vi "Field_Sweep_AMI.vi"   [LabVIEW 2016]
uses:
  Global/Global Variables/global.vi
  Global/Global Variables/Data_Display_global.vi
types:
  T1 = enum16{"", "RAMPING", "HOLDING", "PAUSED", "MANUAL UP", "MANUAL DOWN", "ZEROING CURRENT", "QUENCH DETECTED", "HEATING SWITCH", "AT ZER0", "COOLING SWITCH"}
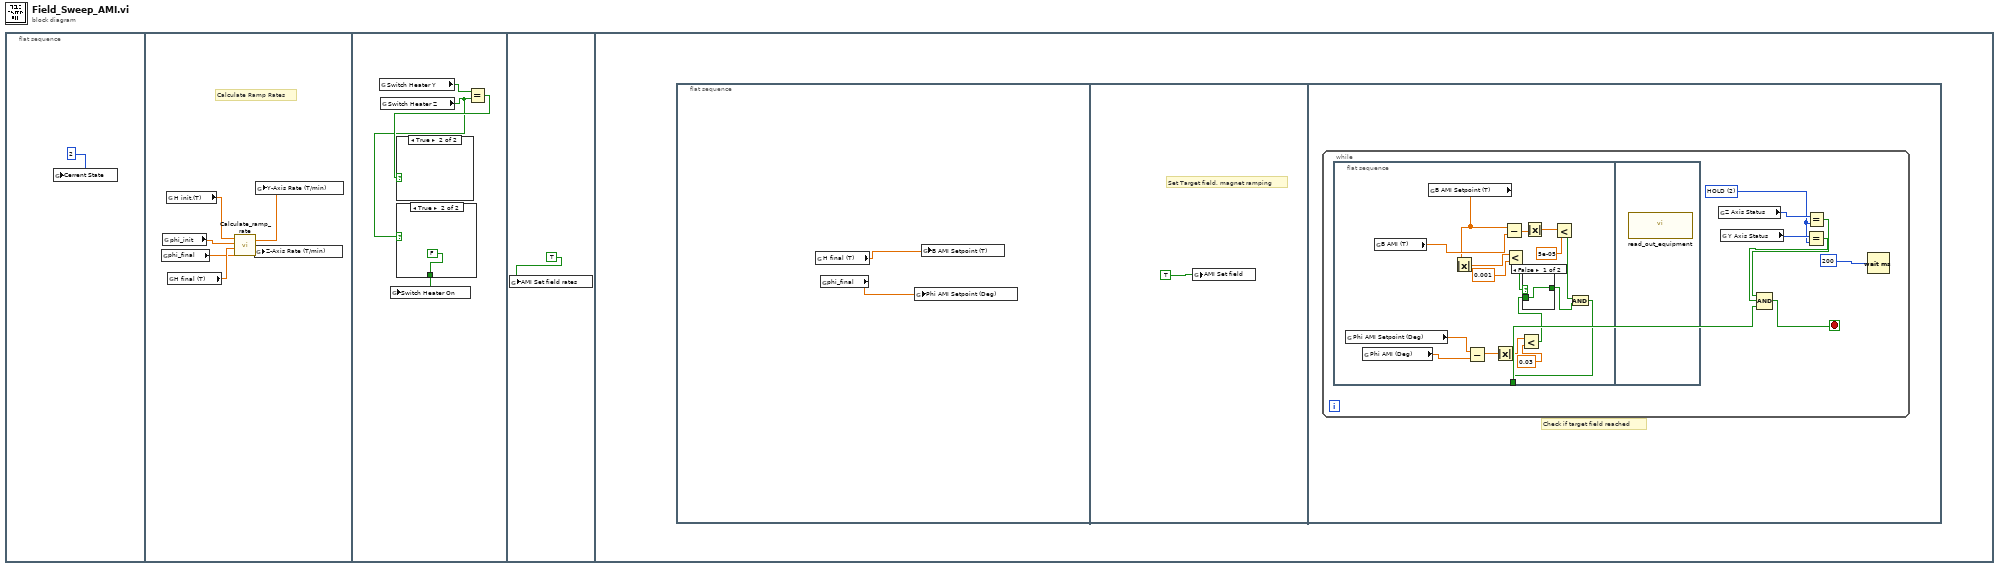
[diagram p0: block diagram]
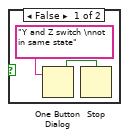
[diagram p2: hidden frame]
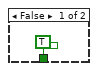
[diagram p3: hidden frame]
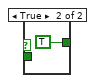
[diagram p4: hidden frame]
diagram:
  n1 = flat-sequence {
    frame #0 {
      n2 = global write "global.vi" "Cerrent State"(2) -> ()
    }
    frame #1 {
      # "Calculate Ramp Rates"
      n3 = global read "global.vi" "phi_final"() -> (w2:dbl)
      n4 = global read "global.vi" "phi_init"() -> (w3:dbl)
      n5 = global read "global.vi" "H init.(T)"() -> (w4:dbl)
      n6 = global read "global.vi" "H final (T)"() -> (w5:dbl)
      n7 = call "Calculate_ramp_rate.vi"("Phi (Deg)"=w2, "H_final (T)"=w5, "Phi_init (Deg)"=w3, "H_init (T)"=w4) -> ("Z-Ramp"=w6:dbl, "Y-Ramp"=w7:dbl)  [unwired: 2 in]
      n8 = global write "Data_Display_global.vi" "Z-Axis Rate (T/min)"(w6) -> ()
      n9 = global write "Data_Display_global.vi" "Y-Axis Rate (T/min)"(w7) -> ()
    }
    frame #2 {
      n10 = global read "Data_Display_global.vi" "Switch Heater Y"() -> (w10:bool)
      n11 = global read "Data_Display_global.vi" "Switch Heater Z"() -> (w8:bool)
      n12 = case shown="True" w8 {
        tunnel: [TRUE FALSE] -> w11
        frame False {
        }
        frame True {
        }
      }
      n13 = global write "Data_Display_global.vi" "Switch Heater On"(w11) -> ()
      n14 = Equal?(x=w10, y=w8) -> (x = y?=w9:bool)
      n15 = case shown="True" w9 {
        frame False {
          n16 = One Button Dialog(message="Y and Z switch \nnot in same state") -> (true=w12:bool)  [unwired: 1 in]
          n17 = Stop(stop? (T)=w12) -> ()
        }
        frame True {
        }
      }
    }
    frame #3 {
      n18 = global write "Data_Display_global.vi" "AMI Set field rates"(TRUE) -> ()
    }
    frame #4 {
      n19 = flat-sequence {
        frame #0 {
          n20 = global read "global.vi" "H final (T)"() -> (w18:dbl)
          n21 = global read "global.vi" "phi_final"() -> (w17:dbl)
          n22 = global write "Data_Display_global.vi" "Phi AMI Setpoint (Deg)"(w17) -> ()
          n23 = global write "Data_Display_global.vi" "B AMI Setpoint (T)"(w18) -> ()
        }
        frame #1 {
          # "Set Target field, magnet ramping"
          n24 = global write "Data_Display_global.vi" "AMI Set field"(TRUE) -> ()
        }
        frame #2 {
          # "Check if target field reached"
          n25 = while {
            stop <- w21 stop-if-true
            w20 = u16 2 items=["RAMP"=1, "HOLD"=2, "Paused"=3, "Manual Up"=4, "Manual Down"=5, "Zeroing Current"=6, "Quench Detected"=7, "At Zero"=8, "Heating Switch"=9, "Cooling Switch "=10] ("Ramping Mode")
            n26 = flat-sequence {
              tunnel: [w34] -> w22
              frame #0 {
                n27 = global read "Data_Display_global.vi" "Phi AMI Setpoint (Deg)"() -> (w37:dbl)
                n28 = global read "Data_Display_global.vi" "Phi AMI (Deg)"() -> (w36:dbl)
                n29 = global read "Data_Display_global.vi" "B AMI (T)"() -> (w41:dbl)
                n30 = global read "Data_Display_global.vi" "B AMI Setpoint (T)"() -> (w30:dbl)
                n31 = Absolute Value(x=w30) -> (abs(x)=w33:dbl)
                n32 = Subtract(x=w37, y=w36) -> (x-y=w38:dbl)
                n33 = Absolute Value(x=w38) -> (abs(x)=w39:dbl)
                n34 = Subtract(x=w30, y=w41) -> (x-y=w43:dbl)
                n35 = Less?(x=w33, y=0.001) -> (x < y?=w31:bool)
                n36 = Less?(x=w39, y=0.03) -> (x < y?=w29:bool)
                n37 = case shown="False" w31 {
                  tunnel: [w45 TRUE] -> w28
                  tunnel: w29 -> [w45 _]
                  frame False {
                  }
                  frame True {
                  }
                }
                n38 = Absolute Value(x=w43) -> (abs(x)=w42:dbl)
                n39 = Less?(x=w42, y=5e-05) -> (x < y?=w35:bool)
                n40 = And(x=w35, y=w28) -> (x .and. y?=w34:bool)
              }
              frame #1 {
                n41 = call "read_out_equipment.vi"() -> ()  [unwired: 1 in]
              }
            }
            n42 = global read "Data_Display_global.vi" "Z Axis Status"() -> (w26:T1)
            n43 = global read "Data_Display_global.vi" "Y Axis Status"() -> (w25:T1)
            n44 = Equal?(x=w25, y=w20) -> (x = y?=w23:bool)
            n45 = Equal?(x=w26, y=w20) -> (x = y?=w24:bool)
            n46 = Compound Arithmetic op=AND(w24, w23, w22) -> (w21:bool)
            n47 = Wait (ms)(milliseconds to wait=200) -> ()  [unwired: 1 out]
          }
        }
      }
    }
  }
